vi "Command Robot.vi"(11 "all rows":dbl[][](array[numeric])) -> ()   [LabVIEW 2020]
uses:
  Framework/Robot Global Data.vi
panel:
  out "Wheel":dbl
  out "Throtle":dbl
  out "Intake Arm Down":bool
  out "Intake Arm Up":bool
  out "Intake":bool
  out "Shooter":bool
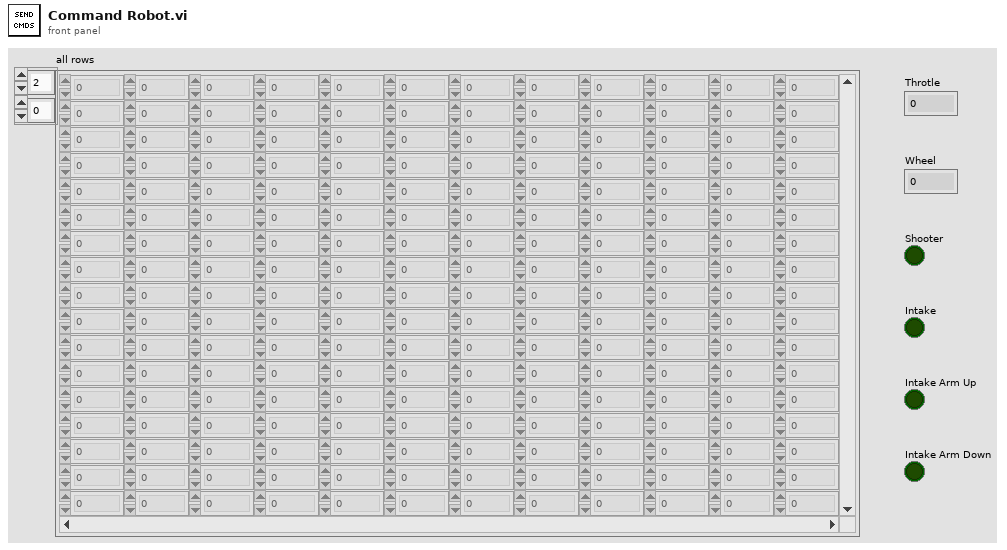
[diagram p1: front panel]
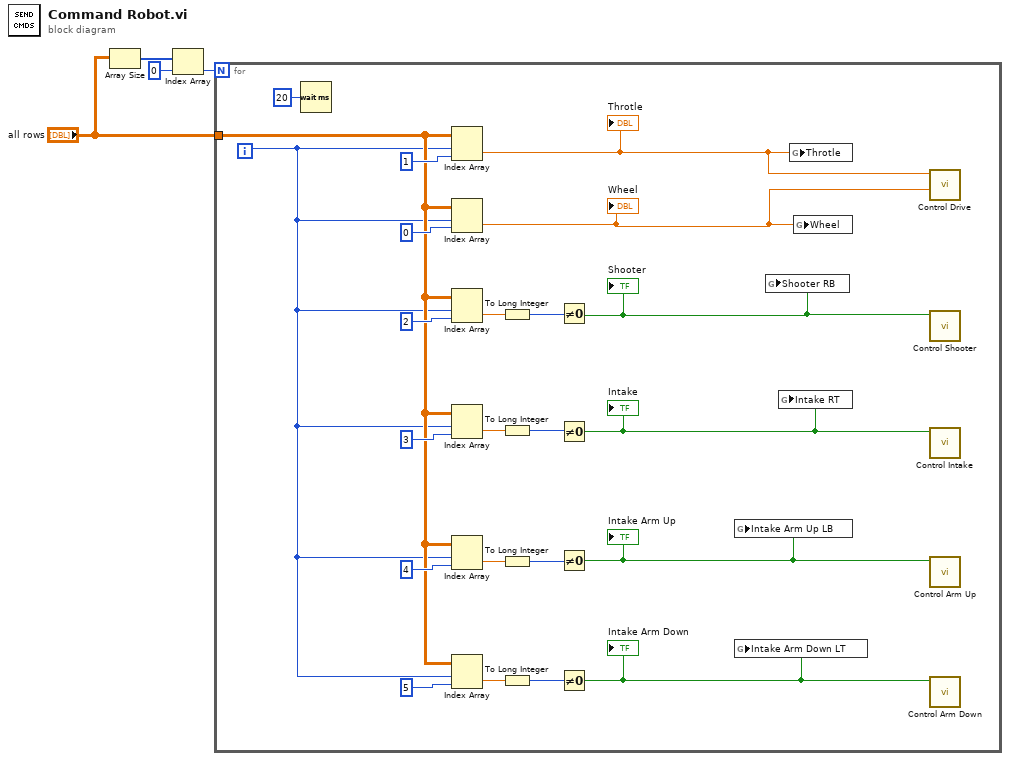
[diagram p0: block diagram]
diagram:
  n1 = Array Size(array="all rows") -> (size(s)=w2:i32[])
  n2 = Index Array(array=w2, index=0) -> (element=w1:i32)
  n3 = for {
    N: w1 -> [_]
    tunnel: "all rows" -> [w17]
    i -> [w16]
    n4 = Wait (ms)(milliseconds to wait=u32 20) -> ()  [unwired: 1 out]
    n5 = Index Array(array=w17, index (row)=w16, index (col)=1 ("disabled index (col)")) -> (element=w6:dbl)
    "Throtle" <- w6
    n6 = Index Array(array=w17, index (row)=w16, index (col)=0 ("disabled index (col)")) -> (element=w5:dbl)
    "Wheel" <- w5
    n7 = Index Array(array=w17, index (row)=w16, index (col)=2 ("disabled index (col)")) -> (element=w21:dbl)
    n8 = Index Array(array=w17, index (row)=w16, index (col)=3 ("disabled index (col)")) -> (element=w23:dbl)
    n9 = Index Array(array=w17, index (row)=w16, index (col)=4 ("disabled index (col)")) -> (element=w25:dbl)
    n10 = Index Array(array=w17, index (row)=w16, index (col)=5 ("disabled index (col)")) -> (element=w27:dbl)
    n11 = To Long Integer(number=w21) -> (32bit integer=w15:i32)
    n12 = To Long Integer(number=w23) -> (32bit integer=w14:i32)
    n13 = To Long Integer(number=w25) -> (32bit integer=w13:i32)
    n14 = To Long Integer(number=w27) -> (32bit integer=w12:i32)
    n15 = Not Equal To 0?(x=w15) -> (x != 0?=w10:bool)
    "Shooter" <- w10
    n16 = Not Equal To 0?(x=w14) -> (x != 0?=w9:bool)
    "Intake" <- w9
    n17 = Not Equal To 0?(x=w13) -> (x != 0?=w8:bool)
    "Intake Arm Up" <- w8
    n18 = Not Equal To 0?(x=w12) -> (x != 0?=w7:bool)
    "Intake Arm Down" <- w7
    n19 = global write "Robot Global Data.vi" "Intake Arm Up LB"(w8) -> ()
    n20 = global write "Robot Global Data.vi" "Intake Arm Down LT"(w7) -> ()
    n21 = global write "Robot Global Data.vi" "Shooter RB"(w10) -> ()
    n22 = global write "Robot Global Data.vi" "Intake RT"(w9) -> ()
    n23 = global write "Robot Global Data.vi" "Throtle"(w6) -> ()
    n24 = global write "Robot Global Data.vi" "Wheel"(w5) -> ()
    n25 = call "Control Drive.vi"("X-DriveAuto"=w5, "Y-DriveAuto"=w6) -> ()  [unwired: 10 in]
    n26 = call "Control Shooter.vi"("Avoid Race Condition"=w10) -> ()  [unwired: 11 in]
    n27 = call "Control Intake.vi"("Avoid Race Condition"=w9) -> ()  [unwired: 11 in]
    n28 = call "Control Arm Up.vi"("Avoid Race Condition"=w8) -> ()  [unwired: 11 in]
    n29 = call "Control Arm Down.vi"("Avoid Race Condition"=w7) -> ()  [unwired: 11 in]
  }
